vi "MoveZ_stepwise.vi"(0 "Z":dbl=60.0, 1 "Zspeed":dbl=25.0, 3 "error in (no error)":errorcluster) -> (7 "MoveZ":string, 8 "controller out":refnum<k24>)   [LabVIEW 2019]
uses:
  C:/Users/TTUHEP/Documents/LabVIEW/Other Models/2010/Bin/Aerotech.A3200.dll
  Other Models/2010/Bin/Aerotech.A3200.dll
panel:
  out "Switch1 2":bool
  out "error out":errorcluster
  # "Move along Z, abs coordinates, with speed v mm/s"
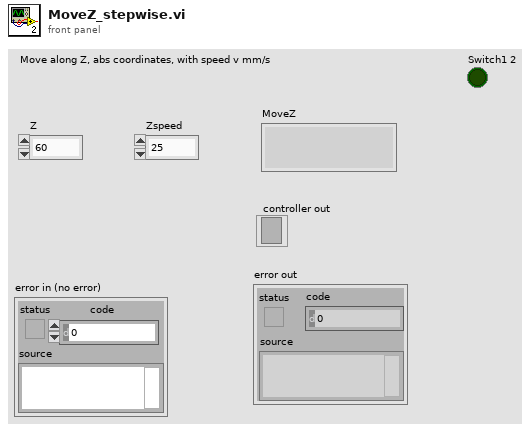
[diagram p1: front panel]
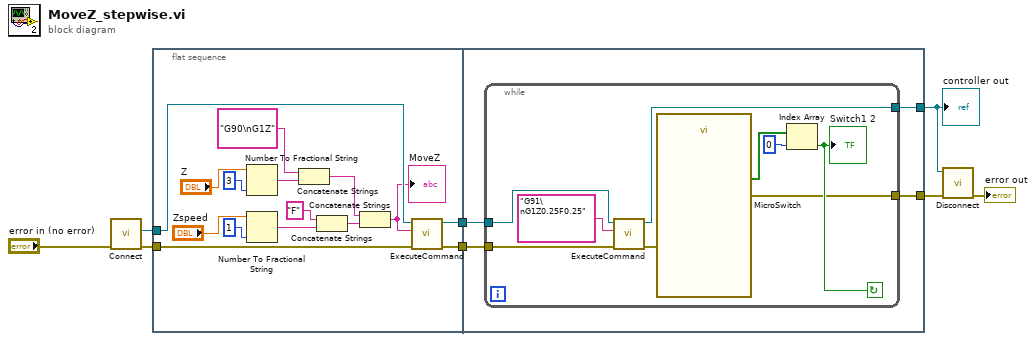
[diagram p0: block diagram]
diagram:
  n1 = call "Connect.vi"("error in (no error)"="error in (no error)") -> ("error out"=w7:errorcluster, "controller"=w6:refnum<k24>)  [unwired: 9 in]
  n2 = flat-sequence {
    tunnel: w7 -> [w23]
    tunnel: w6 -> [w22]
    tunnel: [w21] -> w5
    tunnel: [w20] -> w4
    tunnel: w5 -> [w27]
    tunnel: w4 -> [w26]
    tunnel: [w25] -> w2
    tunnel: [w24] -> w1
    frame #0 {
      n3 = Number To Fractional String(number="Z", precision (6)=i16 3) -> (F-format string=w15:string)  [unwired: 2 in]
      n4 = Number To Fractional String(number="Zspeed", precision (6)=i16 1) -> (F-format string=w18:string)  [unwired: 2 in]
      n5 = Concatenate Strings("G90\nG1Z", w15) -> (w16:string)
      n6 = Concatenate Strings("F" ("string"), w18) -> (w19:string)
      n7 = Concatenate Strings(w16, w19) -> (w9:string)
      "MoveZ" <- w9
      n8 = call "ExecuteCommand.vi"("error in (no error)"=w23, "Command Code"=w9, "controller in"=w22) -> ("error out"=w20:errorcluster, "controller out"=w21:refnum<k24>)  [unwired: 6 in, 1 out]
    }
    frame #1 {
      n9 = while {
        tunnel: w27 -> [w36]
        tunnel: w26 -> [w35]
        tunnel: [w29] -> w25
        tunnel: [w33] -> w24
        stop <- w31 continue-if-true
        n10 = call "ExecuteCommand.vi"("error in (no error)"=w35, "Command Code"="G91\nG1Z0.25F0.25", "controller in"=w36) -> ("error out"=w30:errorcluster, "controller out"=w33:refnum<k24>)  [unwired: 6 in, 1 out]
        n11 = call "MicroSwitch"("error in"=w30) -> ("data"=w28:bool[], "error out"=w29:errorcluster)  [unwired: 16 in, 1 out]
        n12 = Index Array(array=w28, index=0) -> (element=w31:bool)
        "Switch1 2" <- w31
      }
    }
  }
  n13 = call "Disconnect.vi"("error in (no error)"=w2, "controller"=w1) -> ("error out"=→"error out":errorcluster)  [unwired: 9 in]
  "controller out" <- w1
